vi "WriteSettings.vi"(8 "error in (no error)":errorcluster, 10 "Settings":T1={"ipaddress"="192.168.0.254", "Position"={"Axis 1"={"Value"=0.0, "Min"=0.0, "Max"=2.9, "StepSize"=0.001, "Tolerance"=0.0001, "ValueActual"=0.0}, "Axis 2"={"Value"=0.0, "Min"=0.0, "Max"=2.9, "StepSize"=0.001, "Tolerance"=0.0001, "ValueActual"=0.0}, "Axis 3"={"Value"=0.0, "Min"=0.0, "Max"=2.9, "StepSize"=0.001, "Tolerance"=0.0001, "ValueActual"=0.0}, "Axis 4"={"Value"=0.0, "Min"=0.0, "Max"=2.9, "StepSize"=0.001, "Tolerance"=0.0001, "ValueActual"=0.0}, "Axis 5"={"Value"=0.0, "Min"=0.0, "Max"=2.9, "StepSize"=0.001, "Tolerance"=0.0001, "ValueActual"=0.0}, "Axis 6"={"Value"=0.0, "Min"=0.0, "Max"=2.9, "StepSize"=0.001, "Tolerance"=0.0001, "ValueActual"=0.0}}, "PositionerName"={"Axis 1"="", "Axis 2"="", "Axis 3"="", "Axis 4"="", "Axis 5"="", "Axis 6"=""}, "FirstMoveSubtract"={"Axis 1"={"Value"=0.0, "Min"=0.0, "Max"=2.9, "StepSize"=0.001, "Tolerance"=0.0001, "ValueActual"=0.0}, "Axis 2"={"Value"=0.0, "Min"=0.0, "Max"=2.9, "StepSize"=0.001, "Tolerance"=0.0001, "ValueActual"=0.0}, "Axis 3"={"Value"=0.0, "Min"=0.0, "Max"=2.9, "StepSize"=0.001, "Tolerance"=0.0001, "ValueActual"=0.0}, "Axis 4"={"Value"=0.0, "Min"=0.0, "Max"=2.9, "StepSize"=0.001, "Tolerance"=0.0001, "ValueActual"=0.0}, "Axis 5"={"Value"=0.0, "Min"=0.0, "Max"=2.9, "StepSize"=0.001, "Tolerance"=0.0001, "ValueActual"=0.0}, "Axis 6"={"Value"=0.0, "Min"=0.0, "Max"=2.9, "StepSize"=0.001, "Tolerance"=0.0001, "ValueActual"=0.0}}}, 11 "NewportXPS.lvclass":refnum<class "NewportXPS.lvclass">) -> (0 "error out":errorcluster, 3 "NewportXPS.lvclass 2":refnum<class "NewportXPS.lvclass">)   [LabVIEW 2020, in "NewportXPS.lvclass"]
uses:
  NewportXPS.lvclass
  SettingsTypdef.ctl
  NewportXPS.lvclass/NewportXPS.ctl
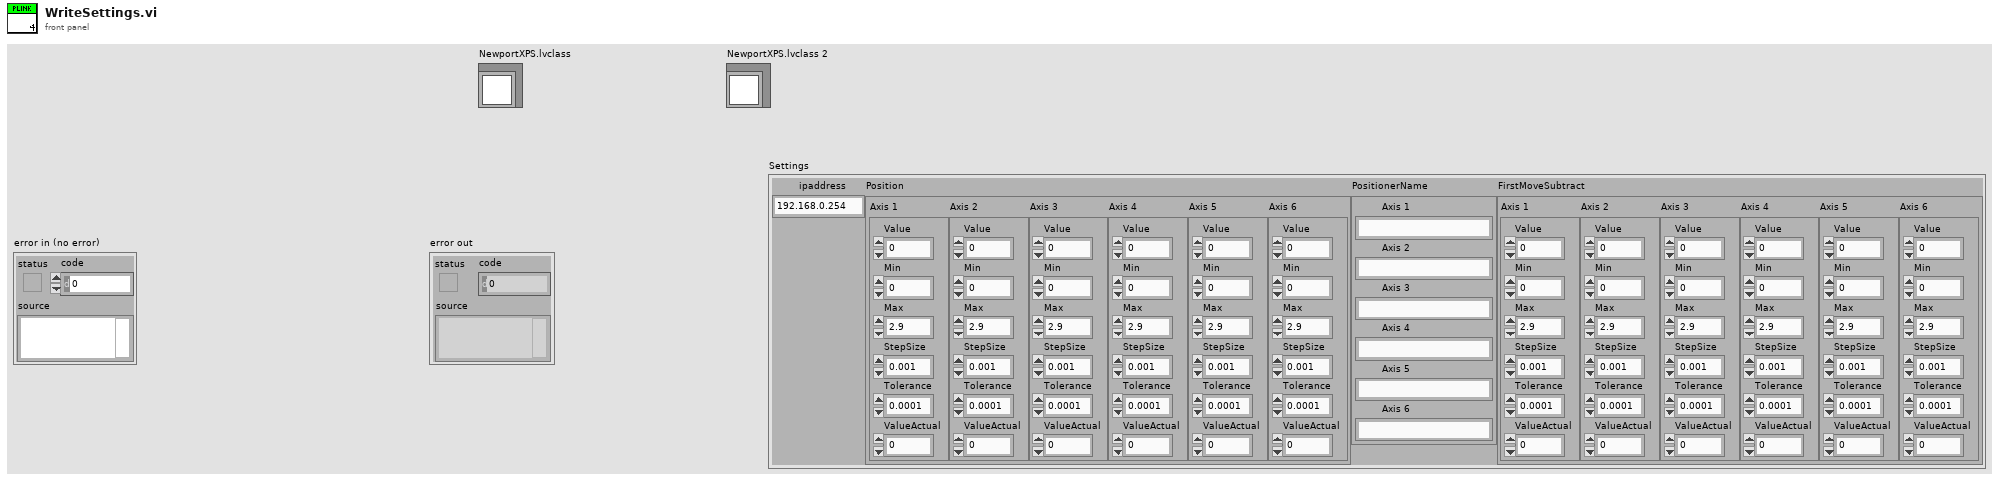
[diagram p1: front panel]
types:
  T1 = typedef "NewportXPS.lvclass/SettingsTypdef.ctl" = cluster{"ipaddress":string, "Position":cluster{"Axis 1":cluster{"Value":dbl, "Min":dbl, "Max":dbl, "StepSize":dbl, "Tolerance":dbl, "ValueActual":dbl}, "Axis 2":cluster{"Value":dbl, "Min":dbl, "Max":dbl, "StepSize":dbl, "Tolerance":dbl, "ValueActual":dbl}, "Axis 3":cluster{"Value":dbl, "Min":dbl, "Max":dbl, "StepSize":dbl, "Tolerance":dbl, "ValueActual":dbl}, "Axis 4":cluster{"Value":dbl, "Min":dbl, "Max":dbl, "StepSize":dbl, "Tolerance":dbl, "ValueActual":dbl}, "Axis 5":cluster{"Value":dbl, "Min":dbl, "Max":dbl, "StepSize":dbl, "Tolerance":dbl, "ValueActual":dbl}, "Axis 6":cluster{"Value":dbl, "Min":dbl, "Max":dbl, "StepSize":dbl, "Tolerance":dbl, "ValueActual":dbl}}, "PositionerName":cluster{"Axis 1":string, "Axis 2":string, "Axis 3":string, "Axis 4":string, "Axis 5":string, "Axis 6":string}, "FirstMoveSubtract":cluster{"Axis 1":cluster{"Value":dbl, "Min":dbl, "Max":dbl, "StepSize":dbl, "Tolerance":dbl, "ValueActual":dbl}, "Axis 2":cluster{"Value":dbl, "Min":dbl, "Max":dbl, "StepSize":dbl, "Tolerance":dbl, "ValueActual":dbl}, "Axis 3":cluster{"Value":dbl, "Min":dbl, "Max":dbl, "StepSize":dbl, "Tolerance":dbl, "ValueActual":dbl}, "Axis 4":cluster{"Value":dbl, "Min":dbl, "Max":dbl, "StepSize":dbl, "Tolerance":dbl, "ValueActual":dbl}, "Axis 5":cluster{"Value":dbl, "Min":dbl, "Max":dbl, "StepSize":dbl, "Tolerance":dbl, "ValueActual":dbl}, "Axis 6":cluster{"Value":dbl, "Min":dbl, "Max":dbl, "StepSize":dbl, "Tolerance":dbl, "ValueActual":dbl}}}
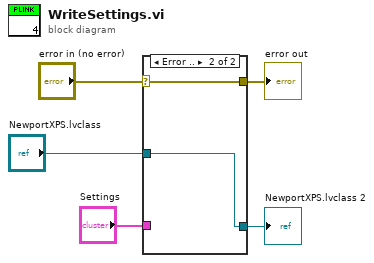
[diagram p0: block diagram]
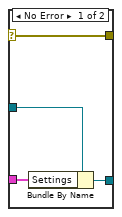
[diagram p2: hidden frame]
diagram:
  n1 = case shown="Error .." "error in (no error)" {
    selector: "error in (no error)" -> [w9 w11]
    tunnel: "NewportXPS.lvclass" -> [w8 w10]
    tunnel: [w9 w11] -> w4
    tunnel: [w7 w10] -> w2
    tunnel: "Settings" -> [w6 _]
    frame No Error {
      n2 = Bundle By Name(cluster=w8, "Settings"=w6) -> (w7:refnum<class "NewportXPS.lvclass">)
    }
    frame Error {
    }
  }
  "NewportXPS.lvclass 2" <- w2
  "error out" <- w4
